vi "Read Incoming Frame.vi"(8 "error in (no error)":errorcluster, 9 "timeout (1000 ms)":i32=1000, 11 "Connection.TCP":refnum<class "Connection.WS.lvclass">) -> (0 "error out":errorcluster, 1 "timed out":bool, 2 "Bytes":u8[](array[numeric]) format="%08b", 3 "Connection.TCP":refnum<class "Connection.WS.lvclass">, 4 "connected":bool, 5 "opcode":T1=2 items=["continuation"=0, "text"=1, "binary"=2, "close"=8, "ping"=9, "pong"=10])   [LabVIEW 2013, in "Connection.WS_GOSPL.lvlib" / "Connection.WS.lvclass"]
uses:
  Connection.WS.lvclass
  Websocket Frame Type -- ring.ctl
  Connection/Connection.lvclass
  Connection.TCP/Connection.TCP.lvclass
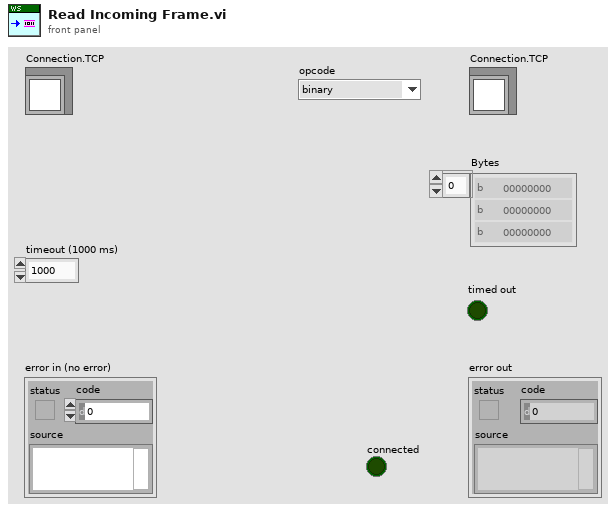
[diagram p1: front panel]
types:
  T1 = typedef "Connection.WS_GOSPL.lvlib/Connection.WS.lvclass/Websocket Frame Type -- ring.ctl" = u8
  T2 = cluster{"state":enum16{"read initial byte", "read payload length", "read extended length", "read mask", "read payload", "end"}, "final-fragment":bool, "opcode":T1, "masked":bool, "extended length":i32, "payload length":i32, "mask":u8[], "payload":u8[]}
  T3 = enum16{"read initial byte", "read payload length", "read extended length", "read mask", "read payload", "end"}
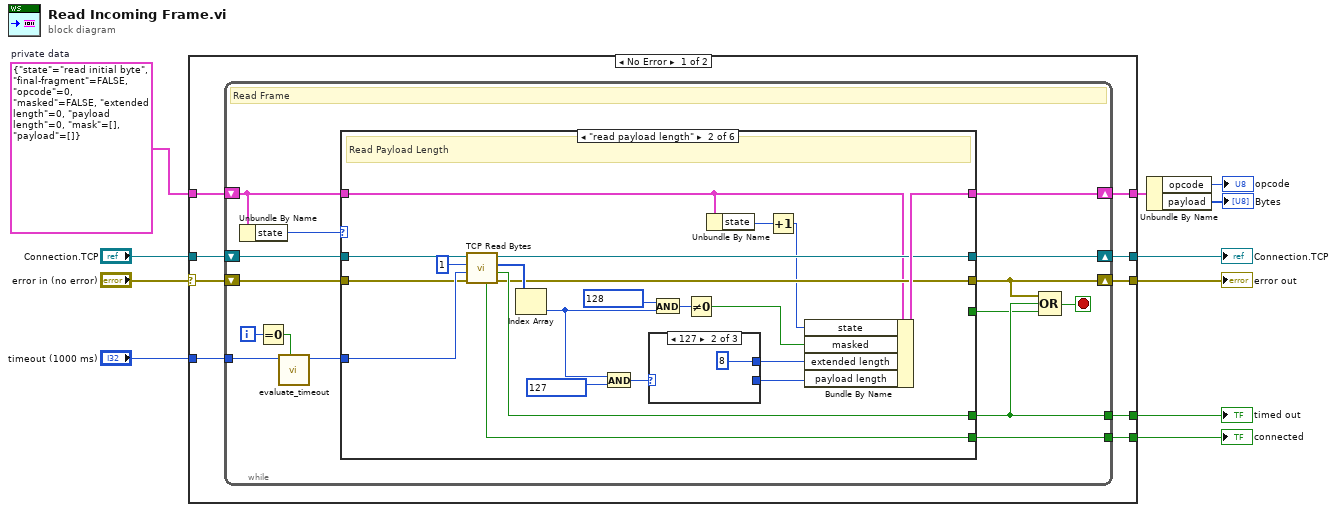
[diagram p0: block diagram]
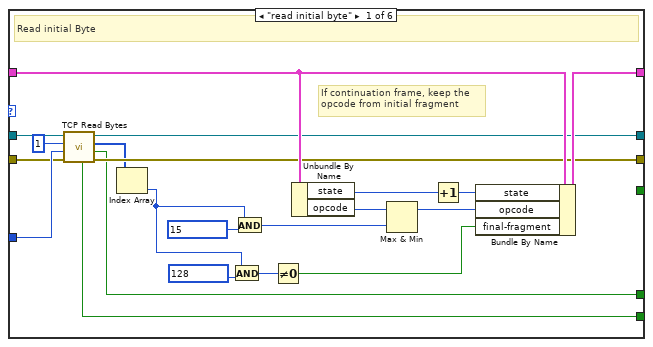
[diagram p2: hidden frame]
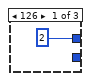
[diagram p3: hidden frame]
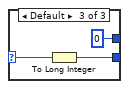
[diagram p4: hidden frame]
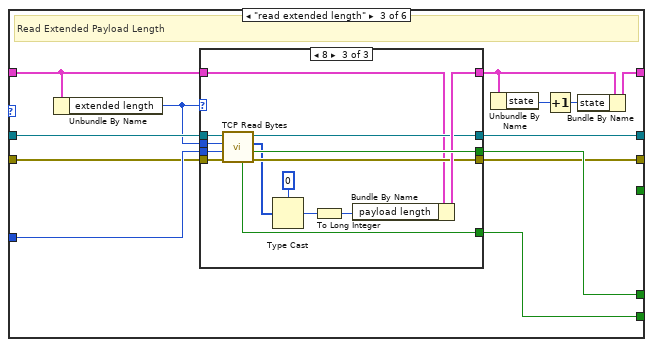
[diagram p5: hidden frame]
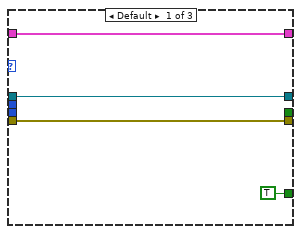
[diagram p6: hidden frame]
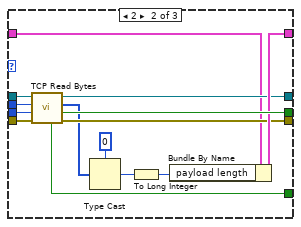
[diagram p7: hidden frame]
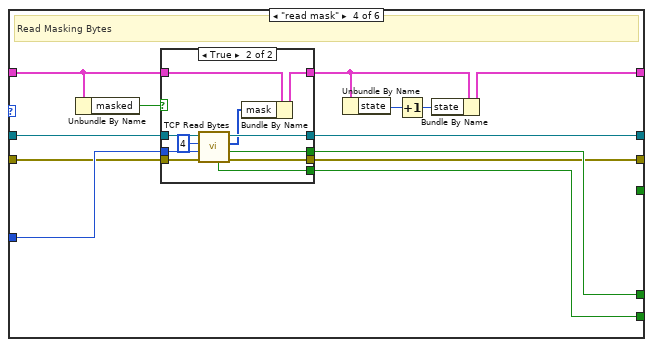
[diagram p8: hidden frame]
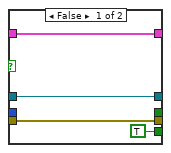
[diagram p9: hidden frame]
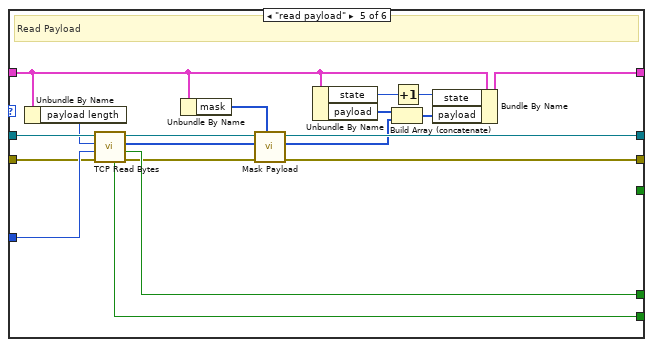
[diagram p10: hidden frame]
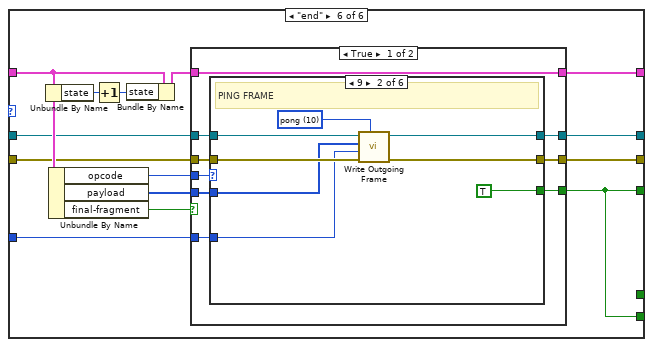
[diagram p11: hidden frame]
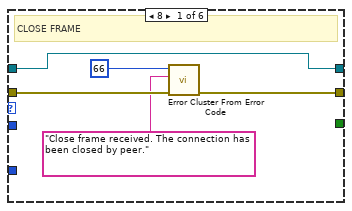
[diagram p12: hidden frame]
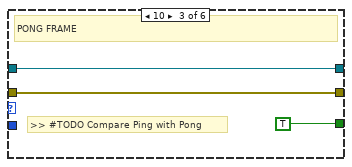
[diagram p13: hidden frame]
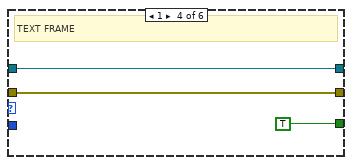
[diagram p14: hidden frame]
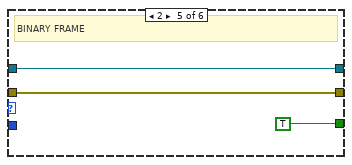
[diagram p15: hidden frame]
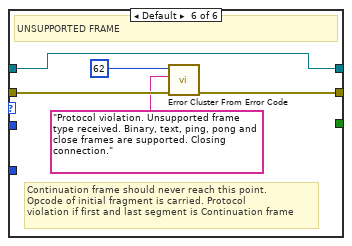
[diagram p16: hidden frame]
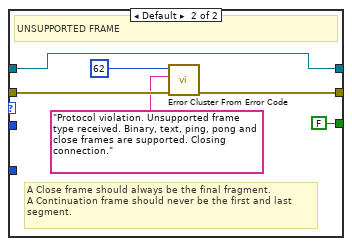
[diagram p18: hidden frame]
diagram:
  w2 = T2 {"state"=enum."read initial byte", "final-fragment"=FALSE, "opcode"=0, "masked"=FALSE, "extended length"=0, "payload length"=0, "mask"=[], "payload"=[]}  # private data
  n1 = case shown="No Error" "error in (no error)" {
    selector: "error in (no error)" -> [w18 w240]
    tunnel: "Connection.TCP" -> [w20 w241]
    tunnel: [w19 w241] -> w8
    tunnel: [w17 w240] -> w7
    tunnel: "timeout (1000 ms)" -> [w16 _]
    tunnel: [w15 _] -> w6
    tunnel: [w14 _] -> w5
    tunnel: w2 -> [w13 _]
    tunnel: [w12 _] -> w3
    frame No Error {
      n2 = while {
        shift-right: [w28] -> w19
        shift-left: w20 -> [w33]
        shift-right: [w30] -> w17
        shift-left: w18 -> [w31]
        tunnel: w16 -> [w34]
        tunnel: [w27] -> w15
        tunnel: [w29] -> w14
        shift-right: [w23] -> w12
        shift-left: w13 -> [w22]
        i -> [w24]
        stop <- w35 stop-if-true
        # "Read Frame"
        n3 = Unbundle By Name(w22) -> ("state"=w21:T3)
        n4 = Equal To 0?(x=w24) -> (x = 0?=w26:bool)
        n5 = call "evaluate_timeout.vi"("reset?"=w26, "timeout (ms)"=w34) -> ("remaining timeout (ms)"=w32:i32)  [unwired: 8 in, 1 out]
        n6 = case shown="\"read payload length\"" w21 {
          tunnel: w33 -> [w44 w77 w95 w140 w172 w183]
          tunnel: w32 -> [w42 w75 w94 w139 w171 w175]
          tunnel: w31 -> [w41 w74 w93 w138 w170 w180]
          tunnel: [w40 w64 w90 w135 w167 w181] -> w30
          tunnel: [w39 w73 w92 w137 w169 _] -> w29
          tunnel: [w37 w65 w91 w136 w168 w182] -> w28
          tunnel: [w38 w57 w83 w128 w156 w176] -> w27
          tunnel: [_ _ _ _ _ w176] -> w25
          tunnel: w22 -> [w51 w59 w89 w134 w165 w186]
          tunnel: [w53 w67 w84 w129 w163 w177] -> w23
          frame "read initial byte" {
            # "If continuation frame, keep the\nopcode from initial fragment"
            # "Read initial Byte"
            n7 = call "TCP Read Bytes.vi"("error in (no error)"=w41, "timeout (1000 ms)"=w42, "bytes to read (100)"=1, "Connection.TCP"=w44) -> ("error out"=w40:errorcluster, "timed out"=w39:bool, "Bytes"=w36:u8[], "Connection.TCP"=w37:refnum<class "Connection.WS.lvclass">, "connected"=w38:bool)  [unwired: 3 in]
            n8 = Index Array(array=w36) -> (element=w48:u8)  [unwired: 1 in]
            n9 = And(x=w48, y=u8 128) -> (x .and. y?=w54:u8)
            n10 = And(x=w48, y=u8 15) -> (x .and. y?=w46:u8)
            n11 = Not Equal To 0?(x=w54) -> (x != 0?=w52:bool)
            n12 = Unbundle By Name(w51) -> ("state"=w50:T3, "opcode"=w47:T1)
            n13 = Max & Min(x=w47, y=w46) -> (max(x,y)=w45:T1)  [unwired: 1 out]
            n14 = Increment(x=w50) -> (x+1=w49:T3)
            n15 = Bundle By Name(cluster=w51, "state"=w49, "opcode"=w45, "final-fragment"=w52) -> (w53:T2)
          }
          frame "read payload length" {
            # "Read Payload Length"
            n16 = call "TCP Read Bytes.vi"("error in (no error)"=w74, "timeout (1000 ms)"=w75, "bytes to read (100)"=1, "Connection.TCP"=w77) -> ("error out"=w64:errorcluster, "timed out"=w73:bool, "Bytes"=w72:u8[], "Connection.TCP"=w65:refnum<class "Connection.WS.lvclass">, "connected"=w57:bool)  [unwired: 3 in]
            n17 = Index Array(array=w72) -> (element=w70:u8)  [unwired: 1 in]
            n18 = And(x=w70, y=u8 127) -> (x .and. y?=w63:u8)
            n19 = case shown="127" w63 {
              selector: w63 -> [_ _ w82]
              tunnel: [_ _ w81] -> w62
              tunnel: [2 8 0] -> w61
              frame 126 {
              }
              frame 127 {
              }
              frame Default {
                n20 = To Long Integer(number=w82) -> (32bit integer=w81:i32)
              }
            }
            n21 = And(x=u8 128, y=w70) -> (x .and. y?=w68:u8)
            n22 = Not Equal To 0?(x=w68) -> (x != 0?=w66:bool)
            n23 = Unbundle By Name(w59) -> ("state"=w60:T3)
            n24 = Increment(x=w60) -> (x+1=w58:T3)
            n25 = Bundle By Name(cluster=w59, "state"=w58, "masked"=w66, "extended length"=w61, "payload length"=w62) -> (w67:T2)
          }
          frame "read extended length" {
            # "Read Extended Payload Length"
            n26 = Unbundle By Name(w89) -> ("extended length"=w88:i32)
            n27 = case shown="8" w88 {
              tunnel: w95 -> [w98 w113 w127]
              tunnel: w94 -> [_ w112 w126]
              tunnel: w93 -> [w97 w111 w125]
              tunnel: [_ w110 w124] -> w92
              tunnel: [w99 w109 w123] -> w85
              tunnel: [w98 w108 w122] -> w91
              tunnel: [w97 w107 w121] -> w90
              tunnel: w89 -> [w99 w105 w119]
              tunnel: w88 -> [_ w104 w118]
              tunnel: [TRUE ("connected") w100 w114] -> w83
              frame Default {
              }
              frame 2 {
                n28 = call "TCP Read Bytes.vi"("error in (no error)"=w111, "timeout (1000 ms)"=w112, "bytes to read (100)"=w104, "Connection.TCP"=w113) -> ("error out"=w107:errorcluster, "timed out"=w110:bool, "Bytes"=w101:u8[], "Connection.TCP"=w108:refnum<class "Connection.WS.lvclass">, "connected"=w100:bool)  [unwired: 3 in]
                n29 = Type Cast(type=u16 0, x=w101) -> (*(type *) &x=w102:u16)
                n30 = To Long Integer(number=w102) -> (32bit integer=w106:i32)
                n31 = Bundle By Name(cluster=w105, "payload length"=w106) -> (w109:T2)
              }
              frame 8 {
                n32 = call "TCP Read Bytes.vi"("error in (no error)"=w125, "timeout (1000 ms)"=w126, "bytes to read (100)"=w118, "Connection.TCP"=w127) -> ("error out"=w121:errorcluster, "timed out"=w124:bool, "Bytes"=w115:u8[], "Connection.TCP"=w122:refnum<class "Connection.WS.lvclass">, "connected"=w114:bool)  [unwired: 3 in]
                n33 = Type Cast(type=u64 0, x=w115) -> (*(type *) &x=w116:u64)
                n34 = To Long Integer(number=w116) -> (32bit integer=w120:i32)
                n35 = Bundle By Name(cluster=w119, "payload length"=w120) -> (w123:T2)
              }
            }
            n36 = Unbundle By Name(w85) -> ("state"=w87:T3)
            n37 = Increment(x=w87) -> (x+1=w86:T3)
            n38 = Bundle By Name(cluster=w85, "state"=w86) -> (w84:T2)
          }
          frame "read mask" {
            # "Read Masking Bytes"
            n39 = Unbundle By Name(w134) -> ("masked"=w133:bool)
            n40 = case shown="True" w133 {
              tunnel: w140 -> [w144 w155]
              tunnel: w139 -> [_ w154]
              tunnel: w138 -> [w143 w153]
              tunnel: [_ w152] -> w137
              tunnel: [w142 w151] -> w130
              tunnel: [w144 w150] -> w136
              tunnel: [w143 w149] -> w135
              tunnel: w134 -> [w142 w148]
              tunnel: [TRUE ("connected") w145] -> w128
              frame False {
              }
              frame True {
                n41 = call "TCP Read Bytes.vi"("error in (no error)"=w153, "timeout (1000 ms)"=w154, "bytes to read (100)"=4, "Connection.TCP"=w155) -> ("error out"=w149:errorcluster, "timed out"=w152:bool, "Bytes"=w146:u8[], "Connection.TCP"=w150:refnum<class "Connection.WS.lvclass">, "connected"=w145:bool)  [unwired: 3 in]
                n42 = Bundle By Name(cluster=w148, "mask"=w146) -> (w151:T2)
              }
            }
            n43 = Unbundle By Name(w130) -> ("state"=w132:T3)
            n44 = Increment(x=w132) -> (x+1=w131:T3)
            n45 = Bundle By Name(cluster=w130, "state"=w131) -> (w129:T2)
          }
          frame "read payload" {
            # "Read Payload"
            n46 = Unbundle By Name(w165) -> ("payload length"=w166:i32)
            n47 = call "TCP Read Bytes.vi"("error in (no error)"=w170, "timeout (1000 ms)"=w171, "bytes to read (100)"=w166, "Connection.TCP"=w172) -> ("error out"=w167:errorcluster, "timed out"=w169:bool, "Bytes"=w164:u8[], "Connection.TCP"=w168:refnum<class "Connection.WS.lvclass">, "connected"=w156:bool)  [unwired: 3 in]
            n48 = Unbundle By Name(w165) -> ("mask"=w157:u8[])
            n49 = call "Mask Payload.vi"("mask"=w157, "Input"=w164) -> ("Output"=w160:u8[])  [unwired: 9 in]
            n50 = Unbundle By Name(w165) -> ("state"=w159:T3, "payload"=w162:u8[])
            n51 = Build Array (concatenate)(w162, w160) -> (w161:u8[])
            n52 = Increment(x=w159) -> (x+1=w158:T3)
            n53 = Bundle By Name(cluster=w165, "state"=w158, "payload"=w161) -> (w163:T2)
          }
          frame "end" {
            n54 = Unbundle By Name(w186) -> ("state"=w185:T3)
            n55 = Unbundle By Name(w186) -> ("opcode"=w173:T1, "payload"=w174:u8[], "final-fragment"=w179:bool)
            n56 = Increment(x=w185) -> (x+1=w184:T3)
            n57 = Bundle By Name(cluster=w186, "state"=w184) -> (w178:T2)
            n58 = case shown="True" w179 {
              tunnel: w173 -> [w195 w231]
              tunnel: w183 -> [w194 w230]
              tunnel: [w193 w229] -> w182
              tunnel: [w192 w228] -> w181
              tunnel: w180 -> [w191 w227]
              tunnel: w178 -> [w190 w226]
              tunnel: [w190 w226] -> w177
              tunnel: [w187 w223] -> w176
              tunnel: w175 -> [w189 w225]
              tunnel: w174 -> [w188 w224]
              frame True {
                n59 = case shown="9" w195 {
                  tunnel: w194 -> [w196 w208 w210 w213 w216 w218]
                  tunnel: [w196 w207 w210 w213 w216 w218] -> w193
                  tunnel: w191 -> [w199 w206 w209 w212 w215 w221]
                  tunnel: [w198 w205 w209 w212 w215 w220] -> w192
                  tunnel: w189 -> [_ w204 _ _ _ _]
                  tunnel: w188 -> [_ w203 _ _ _ _]
                  tunnel: [_ TRUE TRUE TRUE TRUE _] -> w187
                  frame 8 {
                    # "CLOSE FRAME"
                    n60 = call <vilib>:"Error Cluster From Error Code.vi"("error in (no error)"=w199, "error message (\"\")"="Close frame received. The connection has been closed by peer." ("error message (\"\")"), "error code (0)"=66) -> ("error out"=w198:errorcluster)  [unwired: 6 in]
                  }
                  frame 9 {
                    w201 = T1 10 items=["continuation"=0, "text"=1, "binary"=2, "close"=8, "ping"=9, "pong"=10] ("opcode")
                    # "PING FRAME"
                    n61 = call "Write Outgoing Frame.vi"("Frame type"=w201, "error in (no error)"=w206, "timeout ms (2000)"=w204, "Bytes"=w203, "Connection.WS"=w208) -> ("error out"=w205:errorcluster, "Connection.WS"=w207:refnum<class "Connection.WS.lvclass">)  [unwired: 5 in]
                  }
                  frame 10 {
                    # ">> #TODO Compare Ping with Pong"
                    # "PONG FRAME"
                  }
                  frame 1 {
                    # "TEXT FRAME"
                  }
                  frame 2 {
                    # "BINARY FRAME"
                  }
                  frame Default {
                    # "Continuation frame should never reach this point.\nOpcode of initial fragment is carried. Protocol\nviolation if first and last segment is Continuation frame"
                    # "UNSUPPORTED FRAME"
                    n62 = call <vilib>:"Error Cluster From Error Code.vi"("error in (no error)"=w221, "error message (\"\")"="Protocol violation. Unsupported frame type received. Binary, text, ping, pong and close frames are supported. Closing connection." ("error message (\"\")"), "error code (0)"=62) -> ("error out"=w220:errorcluster)  [unwired: 6 in]
                  }
                }
              }
              frame False {
                n63 = case shown="1, 2, 9, 10" w231 {
                  tunnel: w230 -> [w233 w235]
                  tunnel: [w233 w235] -> w229
                  tunnel: w227 -> [w232 w238]
                  tunnel: [w232 w237] -> w228
                  tunnel: w225 -> [_ _]
                  tunnel: w224 -> [_ _]
                  tunnel: [_ FALSE] -> w223
                  frame 1, 2, 9, 10 {
                    # "TEXT\nBINARY\nPING\nPONG"
                    # "SUPPORTED FRAME"
                  }
                  frame Default {
                    # "A Close frame should always be the final fragment.\nA Continuation frame should never be the first and last\nsegment."
                    # "UNSUPPORTED FRAME"
                    n64 = call <vilib>:"Error Cluster From Error Code.vi"("error in (no error)"=w238, "error message (\"\")"="Protocol violation. Unsupported frame type received. Binary, text, ping, pong and close frames are supported. Closing connection." ("error message (\"\")"), "error code (0)"=62) -> ("error out"=w237:errorcluster)  [unwired: 6 in]
                  }
                }
              }
            }
          }
        }
        n65 = Compound Arithmetic op=OR(w30, w29, w25) -> (w35:bool)
      }
    }
    frame Error {
    }
  }
  "error out" <- w7
  "Connection.TCP" <- w8
  "timed out" <- w5
  "connected" <- w6
  n66 = Unbundle By Name(w3) -> ("opcode"=→"opcode":T1, "payload"=→"Bytes":u8[])
